vi "GoToCoordinate.vi"(1 "X PID":T1={"proportional gain (Kc)"=1.0, "integral time (Ti, min)"=0.01, "derivative time (Td, min)"=0.0}, 2 "Face PID Gains":T1={"proportional gain (Kc)"=1.0, "integral time (Ti, min)"=0.01, "derivative time (Td, min)"=0.0} {"derivative time (Td, min)" format="%.3f"; "integral time (Ti, min)" format="%.3f"; "proportional gain (Kc)" format="%.3f"}, 3 "Y PID":T1={"proportional gain (Kc)"=1.0, "integral time (Ti, min)"=0.01, "derivative time (Td, min)"=0.0}, 5 "Target Location":cluster{"X":dbl, "Y":dbl}, 9 "Target Angle (rad)":dbl(knob) scale=3.1416..-3.1416, 11 "error in (no error)":errorcluster, 12 "Position Tolerance":dbl, 14 "Angle Tolerance":dbl) -> (15 "error out":errorcluster)   [LabVIEW 2014]
uses:
  Robot Global Data.vi
  <vilib>/addons/control/pid/pid.llb/PID Control Input Filter (DBL).vi
  <vilib>/addons/control/pid/pid.llb/PID (DBL).vi
  SwerveDriveFace.vi
  <vilib>/addons/control/pid/NI_PID_pid.lvlib
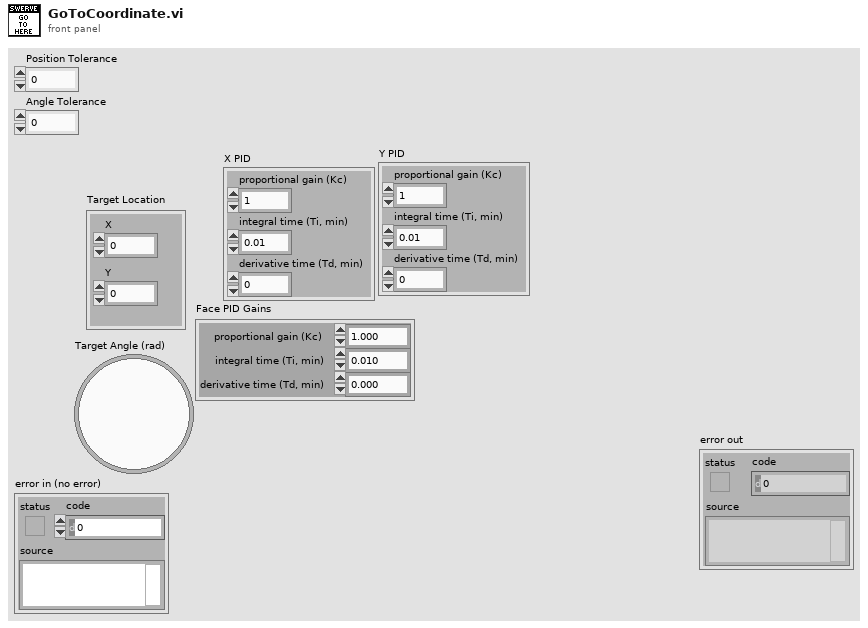
[diagram p1: front panel]
types:
  T1 = cluster{"proportional gain (Kc)":dbl, "integral time (Ti, min)":dbl, "derivative time (Td, min)":dbl}
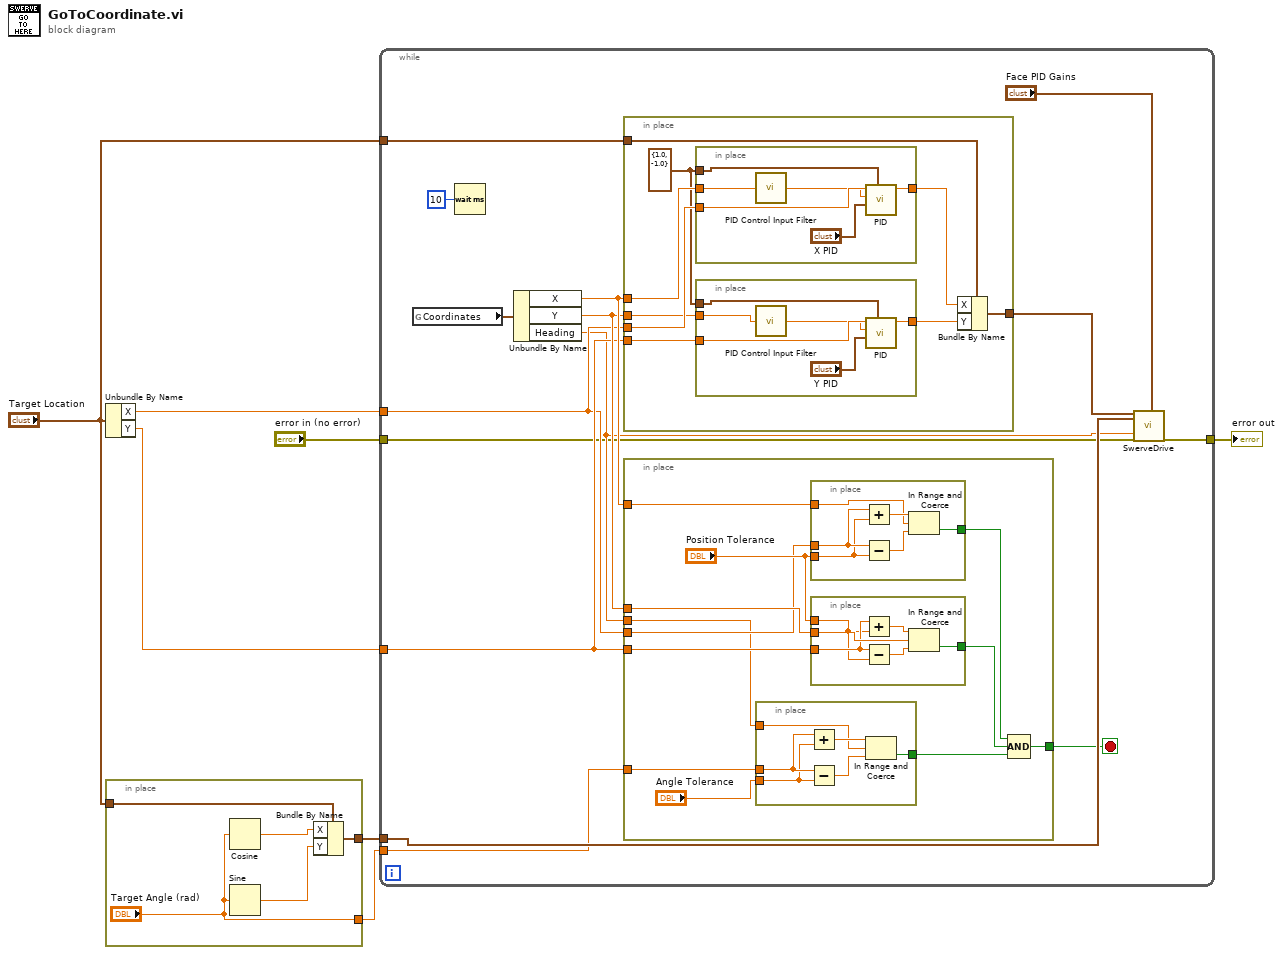
[diagram p0: block diagram]
diagram:
  n1 = Unbundle By Name("Target Location") -> ("X"=w4:dbl, "Y"=w7:dbl)
  n2 = in-place {
    in-place-border: "Target Location" -> [w12]
    in-place-border: [w11] -> w6
    in-place-border: ["Target Angle (rad)"] -> w3
    n3 = Cosine(x="Target Angle (rad)") -> (cos(x)=w8:dbl)
    n4 = Sine(x="Target Angle (rad)") -> (sin(x)=w9:dbl)
    n5 = Bundle By Name(cluster=w12, "X"=w8, "Y"=w9) -> (w11:cluster{"X":dbl, "Y":dbl})
  }
  n6 = while {
    tunnel: w4 -> [w18]
    tunnel: w7 -> [w19]
    tunnel: "Target Location" -> [w24]
    tunnel: w6 -> [w23]
    tunnel: w3 -> [w16]
    tunnel: "error in (no error)" -> [w15]
    tunnel: [w14] -> w1
    stop <- w22 stop-if-true
    n7 = global read "Robot Global Data.vi" "Coordinates"() -> (w27:cluster{"X":dbl, "Y":dbl, "Heading":dbl})
    n8 = Wait (ms)(milliseconds to wait=u32 10) -> ()  [unwired: 1 out]
    n9 = Unbundle By Name(w27) -> ("X"=w21:dbl, "Y"=w20:dbl, "Heading"=w17:dbl)
    n10 = in-place {
      in-place-border: w18 -> [w66]
      in-place-border: w19 -> [w65]
      in-place-border: w21 -> [w64]
      in-place-border: w20 -> [w63]
      in-place-border: [w60] -> w26
      in-place-border: w24 -> [w58]
      w59 = cluster{"output high":dbl, "output low":dbl} {"output high"=1.0, "output low"=-1.0} ("output range")
      n11 = in-place {
        in-place-border: w66 -> [w77]
        in-place-border: w64 -> [w73]
        in-place-border: [w76] -> w62
        in-place-border: w59 -> [w75]
        n12 = call-poly <vilib>:"PID Control Input Filter.vi"("input"=w73) -> ("output"=w74:dbl)  [unwired: 4 in]
        n13 = call-poly <vilib>:"PID.vi"("output range"=w75, "PID gains"="X PID", "process variable"=w74, "setpoint"=w77) -> ("output"=w76:dbl)  [unwired: 6 in, 1 out]
      }
      n14 = in-place {
        in-place-border: w65 -> [w71]
        in-place-border: w63 -> [w68]
        in-place-border: [w70] -> w61
        in-place-border: w59 -> [w69]
        n15 = call-poly <vilib>:"PID Control Input Filter.vi"("input"=w68) -> ("output"=w67:dbl)  [unwired: 4 in]
        n16 = call-poly <vilib>:"PID.vi"("output range"=w69, "PID gains"="Y PID", "process variable"=w67, "setpoint"=w71) -> ("output"=w70:dbl)  [unwired: 6 in, 1 out]
      }
      n17 = Bundle By Name(cluster=w58, "X"=w62, "Y"=w61) -> (w60:cluster{"X":dbl, "Y":dbl})
    }
    n18 = in-place {
      in-place-border: [w39] -> w22
      in-place-border: w21 -> [w37]
      in-place-border: w20 -> [w35]
      in-place-border: w19 -> [w34]
      in-place-border: w18 -> [w33]
      in-place-border: w17 -> [w30]
      in-place-border: w16 -> [w29]
      n19 = in-place {
        in-place-border: [w43] -> w31
        in-place-border: w30 -> [w42]
        in-place-border: w29 -> [w41]
        in-place-border: "Angle Tolerance" -> [w40]
        n20 = Add(x=w41, y=w40) -> (x+y=w45:dbl)
        n21 = Subtract(x=w41, y=w40) -> (x-y=w44:dbl)
        n22 = In Range and Coerce(upper limit=w45, x=w42, lower limit=w44) -> (In Range?=w43:bool)  [unwired: 1 out]
      }
      n23 = in-place {
        in-place-border: [w55] -> w38
        in-place-border: w37 -> [w54]
        in-place-border: w33 -> [w53]
        in-place-border: "Position Tolerance" -> [w52]
        n24 = Add(x=w53, y=w52) -> (x+y=w57:dbl)
        n25 = Subtract(x=w53, y=w52) -> (x-y=w56:dbl)
        n26 = In Range and Coerce(upper limit=w57, x=w54, lower limit=w56) -> (In Range?=w55:bool)  [unwired: 1 out]
      }
      n27 = in-place {
        in-place-border: [w49] -> w32
        in-place-border: w35 -> [w48]
        in-place-border: w34 -> [w47]
        in-place-border: "Position Tolerance" -> [w46]
        n28 = Add(x=w47, y=w46) -> (x+y=w51:dbl)
        n29 = Subtract(x=w47, y=w46) -> (x-y=w50:dbl)
        n30 = In Range and Coerce(upper limit=w51, x=w48, lower limit=w50) -> (In Range?=w49:bool)  [unwired: 1 out]
      }
      n31 = Compound Arithmetic op=AND(w38, w32, w31) -> (w39:bool)
    }
    n32 = call-poly "SwerveDrive.vi"("Strafe Joystick Axes"=w26, "Face Joystick Axes"=w23, "Angle (degrees; 0 = right)"=w17, "error in (no error)"=w15, "Face PID Gains"="Face PID Gains") -> ("error out"=w14:errorcluster)  [unwired: 14 in]
  }
  "error out" <- w1
